vi "力特性 扭矩最大值.vi"(10 "扭矩回":dbl[](array[numeric]), 11 "扭矩去":dbl[](array[numeric])) -> (3 "扭矩最大值":dbl)   [LabVIEW 2015, in "Logging.lvlib"]
uses:
  Logging.lvlib
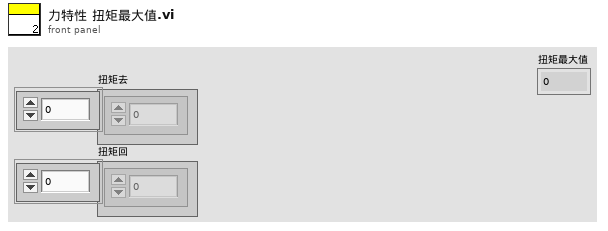
[diagram p1: front panel]
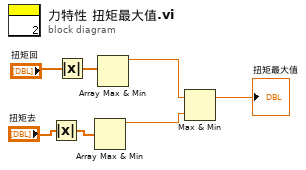
[diagram p0: block diagram]
diagram:
  n1 = Absolute Value(x="扭矩去") -> (abs(x)=w3:dbl[])
  n2 = Absolute Value(x="扭矩回") -> (abs(x)=w1:dbl[])
  n3 = Array Max & Min(array=w3) -> (max value=w6:dbl)  [unwired: 3 out]
  n4 = Array Max & Min(array=w1) -> (max value=w7:dbl)  [unwired: 3 out]
  n5 = Max & Min(x=w7, y=w6) -> (max(x,y)=→"扭矩最大值":dbl)  [unwired: 1 out]
